vi "Write Channel Status for OOB.vi"(8 "error in (no error)":errorcluster, 10 "Channel Status for OOB":T1[](array[typedef]), 11 "CIFChannelMng in":refnum<class "CIFChannelMng.lvclass">) -> (0 "error out":errorcluster, 3 "CIFChannelMng out":refnum<class "CIFChannelMng.lvclass">)   [LabVIEW 2021, in "CIFChannelMng.lvclass"]
uses:
  CIFChannelMng.lvclass
  typedef/Channel List for OOB.ctl
  CIFChannels/Typedef/Direction.ctl
  CIFChannelMng.lvclass/CIFChannelMng.ctl
  CIFChannels/CIFChannels.lvclass
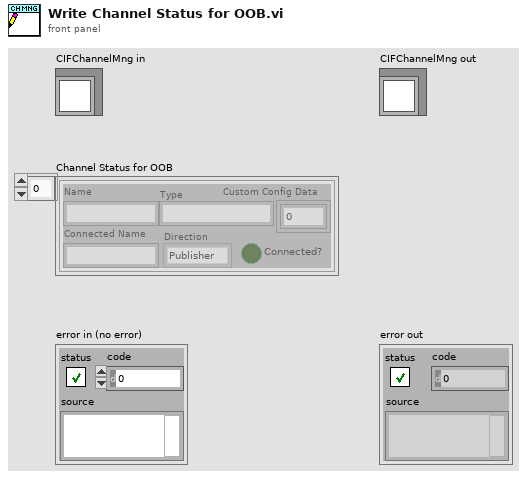
[diagram p1: front panel]
types:
  T1 = typedef "CIFChannelMng.lvclass/Channel List for OOB.ctl" = cluster{"Name":string, "Direction":T2, "Type":string, "Connected?":bool, "Connected Name":string, "Custom Config Data":u8[]}
  T2 = typedef "CIFChannels.lvclass/Direction.ctl" = enum16{"Publisher", "Subscriber"}
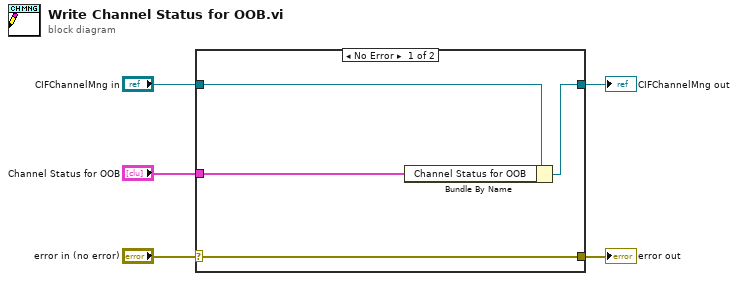
[diagram p0: block diagram]
diagram:
  n1 = case shown="No Error" "error in (no error)" {
    selector: "error in (no error)" -> [w9 w10]
    tunnel: [w9 w10] -> w4
    tunnel: [w7 w11] -> w2
    tunnel: "CIFChannelMng in" -> [w8 w11]
    tunnel: "Channel Status for OOB" -> [w6 _]
    frame No Error {
      n2 = Bundle By Name(cluster=w8, "Channel Status for OOB"=w6) -> (w7:refnum<class "CIFChannelMng.lvclass">)
    }
    frame Error {
    }
  }
  "error out" <- w4
  "CIFChannelMng out" <- w2
